vi "json is equal.vi"(8 "error in (no error)":errorcluster, 9 "json string B":string, 10 "json string A":string, 11 "TestCase in":refnum<class "TestCase.lvclass">) -> (0 "error out":errorcluster, 3 "TestCase out":refnum<class "TestCase.lvclass">)   [LabVIEW 2017, in "ServerTest.lvclass"]
uses:
  ServerTest.lvclass
  <vilib>/addons/_JKI Toolkits/VI Tester/TestCase.llb/TestCase.lvclass
  <vilib>/National Instruments/Variant Data Manipulation/Path API/Read Value at Path(String).vi
  <vilib>/National Instruments/Variant JSON API/Variant JSON API.lvlib
  <vilib>/National Instruments/Variant Data Manipulation/Variant Data Manipulation.lvlib
  <vilib>/Utility/Data Type/NI_Data Type.lvlib
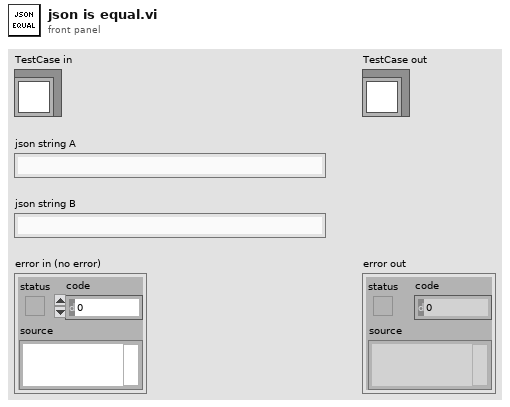
[diagram p1: front panel]
types:
  T1 = typedef "NI_Data Type.lvlib/Data Type.ctl" = enum8{"Invalid Type", "Void", "I8", "I16", "I32", "I64", "U8", "U16", "U32", "U64", "Single Float", "Double Float", "Extended Float", "Single Complex", "Double Complex", "Extended Complex", "Enum U8", "Enum U16", "Enum U32", "Enum U64", "Single Float With Unit", "Double Float With Unit", "Extended Float With Unit", "Single Complex with Unit", "Double Complex with Unit", "Extended Complex with Unit", "Boolean", "String", "Path", "Picture", "Tag", "Array", "Cluster", "Variant", "LV Variant", "Waveform", "Timestamp", "Digital Waveform", "Digital Data", "ExpressData", "Refnum", "External Data", "VI", "Poly VI", "LabVIEW Class Instance", "Fixed Point"}
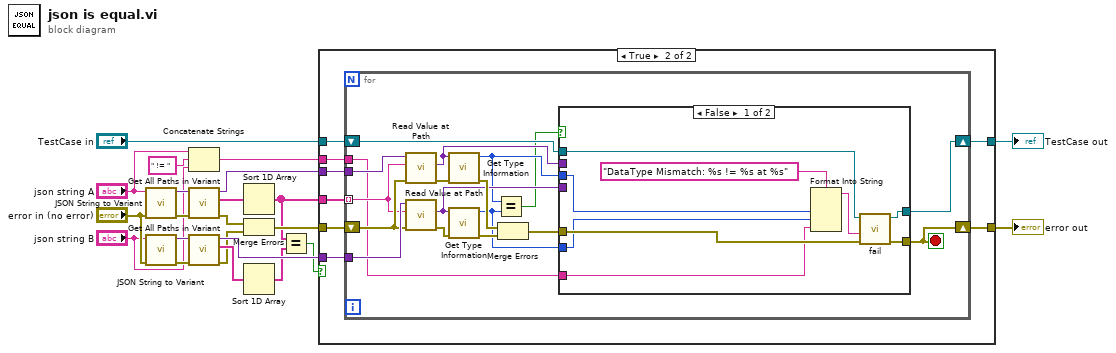
[diagram p0: block diagram]
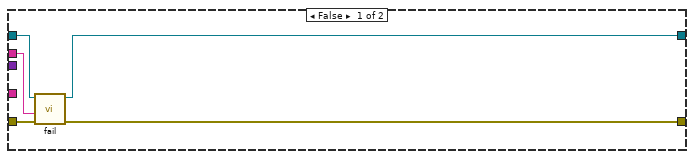
[diagram p2: hidden frame]
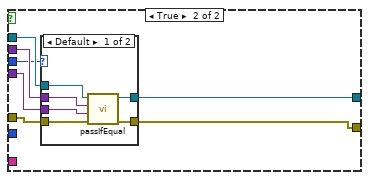
[diagram p3: hidden frame]
diagram:
  n1 = call <vilib>:"JSON String to Variant.vi"("error in (no error)"="error in (no error)", "JSON String"="json string A") -> ("error out"=w8:errorcluster, "Variant out"=w22:variant)  [unwired: 8 in]
  n2 = call <vilib>:"JSON String to Variant.vi"("error in (no error)"="error in (no error)", "JSON String"="json string B") -> ("error out"=w20:errorcluster, "Variant out"=w21:variant)  [unwired: 8 in]
  n3 = Concatenate Strings("json string A", " != " ("string"), "json string B") -> (w4:string)
  n4 = call <vilib>:"Get All Paths in Variant.vi"("error in (no error)"=w8, "Variant in"=w22) -> ("error out"=w13:errorcluster, "Paths out"=w17:string[], "Variant out"=w19:variant)  [unwired: 7 in]
  n5 = call <vilib>:"Get All Paths in Variant.vi"("error in (no error)"=w20, "Variant in"=w21) -> ("error out"=w12:errorcluster, "Paths out"=w16:string[], "Variant out"=w18:variant)  [unwired: 7 in]
  n6 = Sort 1D Array(array=w17) -> (sorted array=w3:string[])
  n7 = Merge Errors(w13, w12) -> (w11:errorcluster)
  n8 = Sort 1D Array(array=w16) -> (sorted array=w2:string[])
  n9 = Equal?(x=w3, y=w2) -> (x = y?=w1:bool)
  n10 = case shown="True" w1 {
    tunnel: w19 -> [_ w35]
    tunnel: w18 -> [_ w34]
    tunnel: "TestCase in" -> [w27 w33]
    tunnel: w11 -> [w26 w32]
    tunnel: [w24 w31] -> w10
    tunnel: [w25 w30] -> w9
    tunnel: w4 -> [w23 w29]
    tunnel: w3 -> [_ w28]
    frame False {
      n11 = call-dynamic "fail.vi"("error in (no error)"=w26, "message (\"\")"=w23, "TestCase in"=w27) -> ("error out"=w25:errorcluster, "TestCase out"=w24:refnum<class "TestCase.lvclass">)  [unwired: 7 in]
    }
    frame True {
      n12 = for {
        tunnel: w35 -> [w53]
        tunnel: w34 -> [w52]
        tunnel: w28 -> [w37] mode=indexing
        shift-right: [w44] -> w31
        shift-left: w33 -> [w50]
        shift-right: [w42] -> w30
        shift-left: w32 -> [w48]
        tunnel: w29 -> [w36]
        stop <- w42 stop-if-true
        n13 = call-poly <vilib>:"Read Value at Path.vi"("error in (no error)"=w48, "Path String"=w37, "Variant in"=w53) -> ("error out"=w43:errorcluster, "Element out"=w49:variant)  [unwired: 6 in, 1 out]
        n14 = call-poly <vilib>:"Read Value at Path.vi"("error in (no error)"=w48, "Path String"=w37, "Variant in"=w52) -> ("error out"=w51:errorcluster, "Element out"=w41:variant)  [unwired: 6 in, 1 out]
        n15 = call <vilib>:"Get Type Information.vi"("error in (no error)"=w43, "Variant"=w49) -> ("error out"=w47:errorcluster, "Type"=w40:T1)  [unwired: 5 in, 3 out]
        n16 = call <vilib>:"Get Type Information.vi"("error in (no error)"=w51, "Variant"=w41) -> ("error out"=w46:errorcluster, "Type"=w38:T1)  [unwired: 5 in, 3 out]
        n17 = Equal?(x=w40, y=w38) -> (x = y?=w39:bool)
        n18 = Merge Errors(w47, w46) -> (w45:errorcluster)
        n19 = case shown="False" w39 {
          tunnel: w50 -> [w62 w69]
          tunnel: w49 -> [_ w68]
          tunnel: w45 -> [w59 w67]
          tunnel: [w61 w66] -> w44
          tunnel: [w60 w65] -> w42
          tunnel: w41 -> [_ w64]
          tunnel: w40 -> [w57 w63]
          tunnel: w38 -> [w56 _]
          tunnel: w36 -> [w54 _]
          frame False {
            n20 = Format Into String(format string="DataType Mismatch: %s != %s at %s" ("custom report message (\"\")"), w57, w56, w54) -> (resulting string=w55:string)  [unwired: 2 in, 1 out]
            n21 = call-dynamic "fail.vi"("error in (no error)"=w59, "message (\"\")"=w55, "TestCase in"=w62) -> ("error out"=w60:errorcluster, "TestCase out"=w61:refnum<class "TestCase.lvclass">)  [unwired: 7 in]
          }
          frame True {
            n22 = case shown="Default" w63 {
              tunnel: w69 -> [w71 w77]
              tunnel: w68 -> [w75 _]
              tunnel: w64 -> [w74 _]
              tunnel: w67 -> [w73 w76]
              tunnel: [w72 w76] -> w65
              tunnel: [w70 w77] -> w66
              frame Default {
                n23 = call-dynamic "passIfEqual.vi"("error in (no error)"=w73, "y"=w74, "x"=w75, "TestCase in"=w71) -> ("error out"=w72:errorcluster, "TestCase out"=w70:refnum<class "TestCase.lvclass">)  [unwired: 6 in]
              }
              frame "Array", "Cluster" {
              }
            }
          }
        }
      }
    }
  }
  "error out" <- w9
  "TestCase out" <- w10
